vi "testTTL_v2.vi"() -> ()   [LabVIEW 2015]
uses:
  <vilib>/DAQmx/write.llb/DAQmx Write (Digital Bool 1Line 1Point).vi
  <vilib>/DAQmx/write.llb/DAQmx Write (Analog Wfm 1Chan NSamp).vi
  <vilib>/DAQmx/miscellaneous.llb/DAQmx Fill In Error Info.vi
  Windows/System32/kernel32.dll
panel:
  out "wait time (ms)":dbl
  out "count 3":u64
  in  "delay (ms)":dbl
  out "DAQ error out":errorcluster
  out "count 4":u64
  out "count 2":u64
  out "count 1":u64
  out "wait end to pulse gen end (ms)":dbl
  out "OEP to wait start (ms)":dbl caption="event rx to pulse gen start (ms)"
  out "time off (s)":dbl
  in  "Stop":bool
  out "level":sgl
  out "time on (s)":dbl
  out "New event":bool
  in  "event channel":u8=1 min=1 max=8
  out "TTL error out":errorcluster
  in  "error in":errorcluster
  in  "port":u16
  # "Timing"
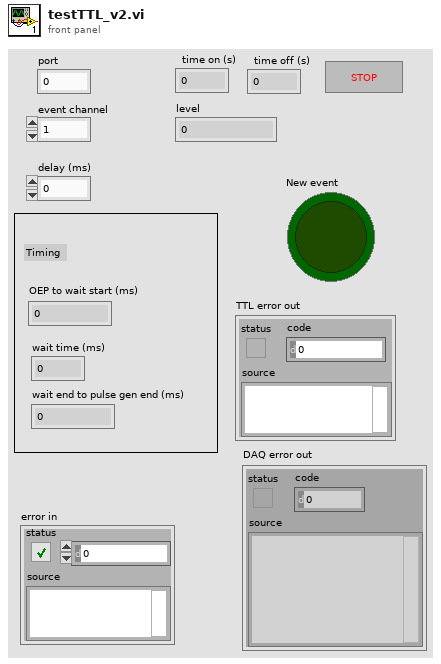
[diagram p1: front panel]
types:
  T1 = enum16{"big-endian, network order", "native, host order", "little-endian"}
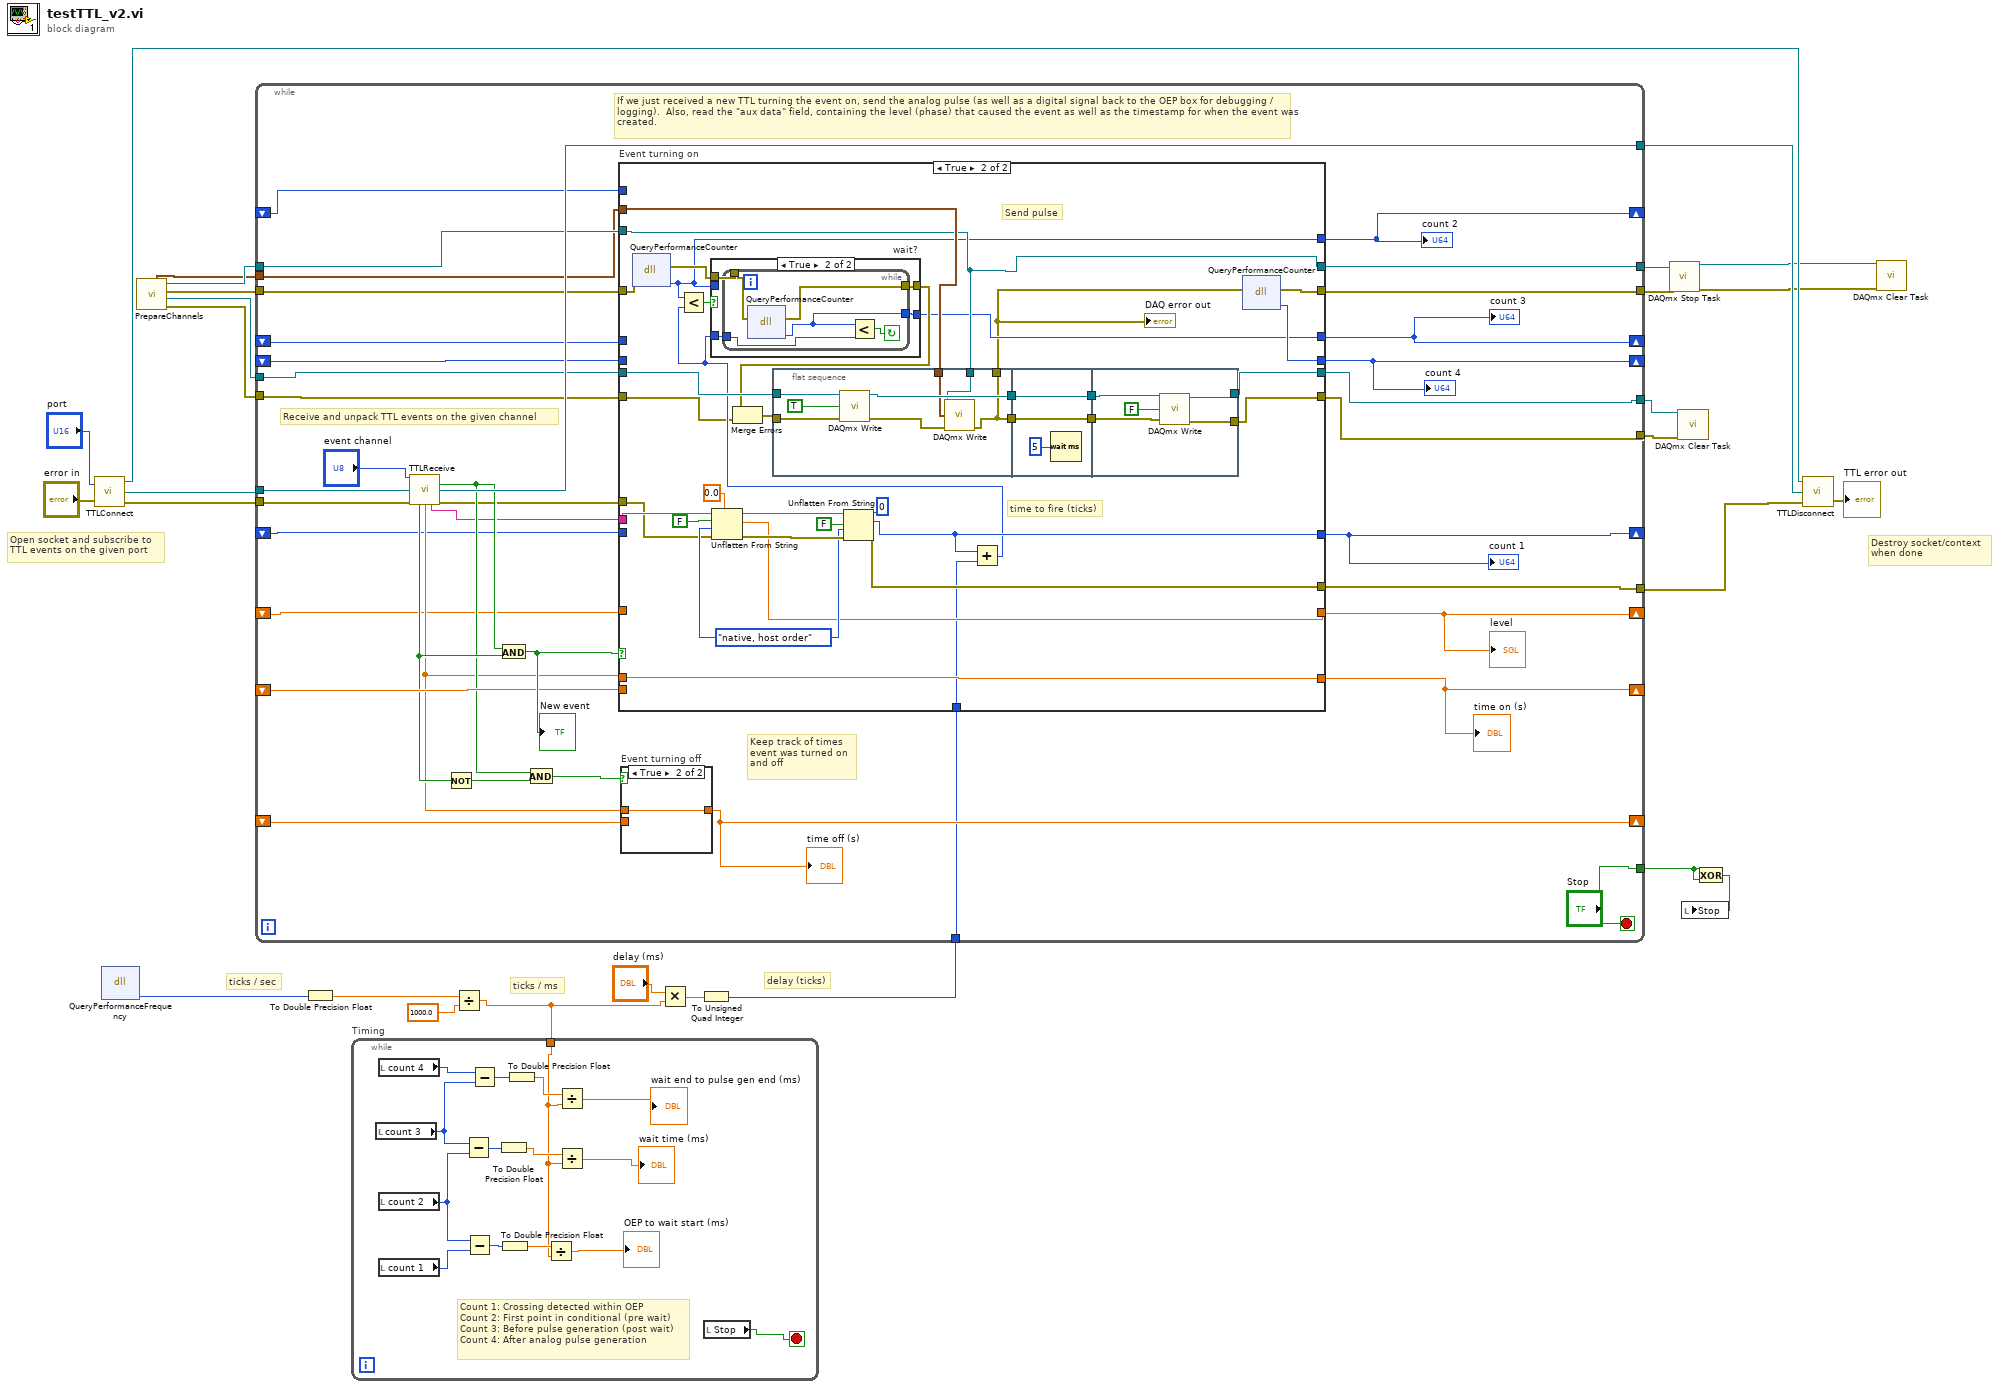
[diagram p0: block diagram]
diagram:
  # "delay (ticks)"
  # "ticks / ms"
  # "ticks / sec"
  # "Open socket and subscribe to\nTTL events on the given port"
  # "Destroy socket/context\nwhen done"
  n1 = call "TTLConnect.vi"("port"="port", "error in"="error in") -> ("context out"=w27:refnum<class "zmq_context.lvclass">, "socket out"=w9:refnum<class "zmq_socket.lvclass">, "error out"=w10:errorcluster)
  n2 = dll-call lib="C:/Windows/System32/kernel32.dll" fn="QueryPerformanceFrequency"() -> ("lpFrequency"=w7:u64)  [unwired: 5 in, 2 out]
  n3 = call "PrepareChannels.vi"() -> ("DO error out"=w21:errorcluster, "DO task out"=w22:refnum<k21>, "AO error out"=w20:errorcluster, "AO task out"=w23:refnum<k21>, "Waveform Graph"=w15:waveform(dbl))  [unwired: 7 in]
  n4 = To Double Precision Float(number=w7) -> (double precision float=w5:dbl)
  n5 = Divide(x=w5, y=1000.0) -> (x/y=w4:dbl)
  n6 = while "Timing" {
    tunnel: w4 -> [w30]
    stop <- w37 stop-if-true
    # "Count 1: Crossing detected within OEP\nCount 2: First point in conditional (pre wait)\nCount 3: Before pulse generation (post wait)\nCount 4: After analog pulse generation"
    n7 = local read "count 3"() -> (w33:u64)
    n8 = local read "count 4"() -> (w43:u64)
    n9 = local read "count 2"() -> (w34:u64)
    n10 = local read "count 1"() -> (w38:u64)
    n11 = Subtract(x=w33, y=w34) -> (x-y=w32:u64)
    n12 = Subtract(x=w34, y=w38) -> (x-y=w41:u64)
    n13 = Subtract(x=w43, y=w33) -> (x-y=w42:u64)
    n14 = To Double Precision Float(number=w32) -> (double precision float=w31:dbl)
    n15 = To Double Precision Float(number=w41) -> (double precision float=w39:dbl)
    n16 = To Double Precision Float(number=w42) -> (double precision float=w40:dbl)
    n17 = Divide(x=w39, y=w30) -> (x/y=→"OEP to wait start (ms)":dbl)
    n18 = Divide(x=w40, y=w30) -> (x/y=→"wait end to pulse gen end (ms)":dbl)
    n19 = Divide(x=w31, y=w30) -> (x/y=→"wait time (ms)":dbl)
    n20 = local read "Stop"() -> (w37:bool)
  }
  n21 = Multiply(x="delay (ms)", y=w4) -> (x*y=w2:dbl)
  n22 = To Unsigned Quad Integer(1:w2) -> (0:w1:u64)
  n23 = while {
    tunnel: w10 -> [w81]
    tunnel: [w55] -> w8
    tunnel: [w80] -> w26
    tunnel: w9 -> [w79]
    shift-right: [w56] -> _
    shift-left: _ -> [w53]
    shift-right: [w65] -> _
    shift-left: _ -> [w64]
    shift-right: [w77] -> _
    shift-left: _ -> [w76]
    shift-right: [w54] -> _
    shift-left: _ -> [w52]
    tunnel: w23 -> [w74]
    tunnel: w22 -> [w72]
    tunnel: w21 -> [w71]
    tunnel: w20 -> [w73]
    shift-right: [w70] -> _
    shift-left: _ -> [w68]
    shift-right: [w69] -> _
    shift-left: _ -> [w67]
    tunnel: [w48] -> w14
    tunnel: [w47] -> w13
    tunnel: [w51] -> w19
    tunnel: [w66] -> w18
    tunnel: ["Stop"] -> w17
    tunnel: w15 -> [w49]
    tunnel: w1 -> [w46]
    shift-right: [w45] -> _
    shift-left: _ -> [w44]
    stop <- "Stop" stop-if-true
    # "If we just received a new TTL turning the event on, send the analog pulse (as well as a digital signal back to the OEP box for debugging / logging).  Also, read the \"aux data\" field, containing the level (phase) that caused the event as well as the timestamp for when the event was created."
    # "Keep track of times\nevent was turned on\nand off"
    # "Receive and unpack TTL events on the given channel"
    n24 = call "TTLReceive.vi"("channel"="event channel", "socket in"=w79, "error in"=w81) -> ("new TTL"=w61:bool, "socket out"=w80:refnum<class "zmq_socket.lvclass">, "event on"=w62:bool, "timestamp (s)"=w59:dbl, "aux data"=w58:string, "error out"=w57:errorcluster)  [unwired: 6 in, 1 out]
    n25 = Not(x=w62) -> (.not. x?=w63:bool)
    n26 = And(x=w61, y=w62) -> (x .and. y?=w75:bool)
    "New event" <- w75
    n27 = And(x=w61, y=w63) -> (x .and. y?=w60:bool)
    n28 = case "Event turning on" shown="True" w75 {
      tunnel: w74 -> [w92 w96]
      tunnel: w73 -> [w91 w126]
      tunnel: [w92 w96] -> w48
      tunnel: [w91 w125] -> w47
      tunnel: w72 -> [w84 w123]
      tunnel: w71 -> [w83 w100]
      tunnel: [w84 w127] -> w51
      tunnel: [w83 w98] -> w66
      tunnel: [w90 w95] -> w70
      tunnel: w68 -> [w90 _]
      tunnel: [w89 w124] -> w69
      tunnel: w67 -> [w89 _]
      tunnel: w59 -> [_ w122]
      tunnel: [w88 w122] -> w65
      tunnel: w64 -> [w88 _]
      tunnel: w58 -> [_ w114]
      tunnel: w57 -> [w85 w111]
      tunnel: [w86 w105] -> w54
      tunnel: [w85 w113] -> w55
      tunnel: [w87 w112] -> w56
      tunnel: w53 -> [w87 _]
      tunnel: w52 -> [w86 _]
      tunnel: w49 -> [_ w97]
      tunnel: w46 -> [_ w106]
      tunnel: [w82 w94] -> w45
      tunnel: w44 -> [w82 _]
      frame False {
      }
      frame True {
        w116 = T1."native, host order" ("byte order (0:big-endian, network order)")
        # "time to fire (ticks)"
        # "Send pulse"
        n29 = dll-call lib="C:/Windows/System32/kernel32.dll" fn="QueryPerformanceCounter" label="QPC"(error in=w126) -> (error out=w103:errorcluster, "lpPerformanceCount"=w95:u64)  [unwired: 4 in, 1 out]
        n30 = Unflatten From String(type=sgl 0.0, binary string=w114, data includes array or string size? (T)=FALSE, byte order (0:big-endian, network order)=w116, error in (no error)=w111) -> (rest of the binary string=w118:string, value=w112:sgl, error out=w119:errorcluster)
        n31 = flat-sequence {
          tunnel: w101 -> [w143]
          tunnel: w123 -> [w145]
          tunnel: [w144] -> w110
          tunnel: [w139] -> w109
          tunnel: w97 -> [w141]
          tunnel: w96 -> [w140]
          tunnel: [w139] -> w93
          tunnel: [w149] -> w108
          tunnel: w110 -> [w149]
          tunnel: [w148] -> w107
          tunnel: w109 -> [w148]
          tunnel: [w152] -> w127
          tunnel: w108 -> [w153]
          tunnel: w107 -> [w151]
          tunnel: [w150] -> w98
          frame #0 {
            n32 = call-poly <vilib>:"DAQmx Write.vi"("task/channels in"=w145, "data"=TRUE, "error in"=w143) -> ("task out"=w144:refnum<k21>, "error out"=w142:errorcluster)  [unwired: 10 in, 1 out]
            n33 = call-poly <vilib>:"DAQmx Write.vi"("task/channels in"=w140, "data"=w141, "error in"=w142) -> ("error out"=w139:errorcluster)  [unwired: 10 in, 2 out]
          }
          frame #1 {
            n34 = Wait (ms)(milliseconds to wait=u32 5) -> ()  [unwired: 1 out]
          }
          frame #2 {
            n35 = call-poly <vilib>:"DAQmx Write.vi"("task/channels in"=w153, "data"=FALSE, "error in"=w151) -> ("task out"=w152:refnum<k21>, "error out"=w150:errorcluster)  [unwired: 10 in, 1 out]
          }
        }
        n36 = Unflatten From String(type=u64 0, binary string=w118, data includes array or string size? (T)=FALSE, byte order (0:big-endian, network order)=w116, error in (no error)=w119) -> (value=w105:u64, error out=w113:errorcluster)  [unwired: 1 out]
        n37 = Add(x=w105, y=w106) -> (x+y=w102:u64)
        n38 = Less?(x=w95, y=w102) -> (x < y?=w104:bool)
        n39 = case "wait?" shown="True" w104 {
          tunnel: w103 -> [w128 w133]
          tunnel: [w128 w132] -> w99
          tunnel: w102 -> [_ w131]
          tunnel: [w129 w130] -> w94
          tunnel: w95 -> [w129 _]
          frame False {
          }
          frame True {
            n40 = while {
              tunnel: w133 -> [w138]
              tunnel: [w137] -> w132
              tunnel: w131 -> [w135]
              tunnel: [w134] -> w130
              stop <- w136 continue-if-true
              n41 = dll-call lib="C:/Windows/System32/kernel32.dll" fn="QueryPerformanceCounter" label="QPC"(error in=w138) -> (error out=w137:errorcluster, "lpPerformanceCount"=w134:u64)  [unwired: 4 in, 1 out]
              n42 = Less?(x=w134, y=w135) -> (x < y?=w136:bool)
            }
          }
        }
        n43 = Merge Errors(w99, w100) -> (w101:errorcluster)
        n44 = dll-call lib="C:/Windows/System32/kernel32.dll" fn="QueryPerformanceCounter"(error in=w93) -> (error out=w125:errorcluster, "lpPerformanceCount"=w124:u64)  [unwired: 4 in, 1 out]
        "DAQ error out" <- w93
      }
    }
    "time on (s)" <- w65
    "level" <- w56
    "count 1" <- w54
    "count 2" <- w70
    "count 4" <- w69
    "count 3" <- w45
    n45 = case "Event turning off" shown="True" w60 {
      tunnel: [w155 w156] -> w77
      tunnel: w76 -> [w155 _]
      tunnel: w59 -> [_ w156]
      frame False {
      }
      frame True {
      }
    }
    "time off (s)" <- w77
  }
  n46 = call <vilib>:"DAQmx Stop Task.vi"("task/channels in"=w14, "error in"=w13) -> ("task out"=w12:refnum<k21>, "error out"=w11:errorcluster)  [unwired: 12 in]
  n47 = call <vilib>:"DAQmx Clear Task.vi"("task in"=w19, "error in"=w18) -> ()  [unwired: 13 in, 1 out]
  n48 = Exclusive Or(1:w17, 2:w17) -> (0:w16:bool)
  n49 = local write "Stop"(w16) -> ()
  n50 = call "TTLDisconnect.vi"("error in"=w8, "socket in"=w26, "context in"=w27) -> ("error out"=→"TTL error out":errorcluster)  [unwired: 1 in]
  n51 = call <vilib>:"DAQmx Clear Task.vi"("task in"=w12, "error in"=w11) -> ()  [unwired: 13 in, 1 out]
